vi "Tear Down TS.vi"(8 "error in (no error)":errorcluster, 11 "LNG Boiling Test Stand in":refnum<class "Water Tunnel Test Stand.lvclass">) -> (0 "error out":errorcluster, 3 "LNG Boiling Test Stand out":refnum<class "Water Tunnel Test Stand.lvclass">)   [LabVIEW 2019, in "Test Stands.lvlib" / "Water Tunnel Test Stand.lvclass"]
uses:
  Water Tunnel Test Stand.lvclass
  Water Tunnel Test Stand.lvclass/Water Tunnel Test Stand.ctl
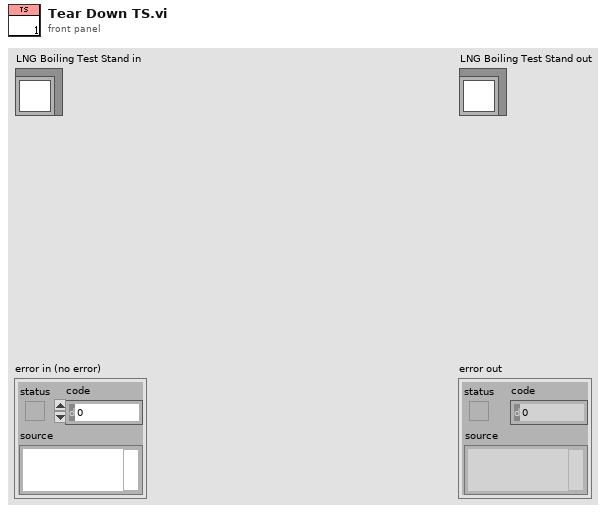
[diagram p1: front panel]
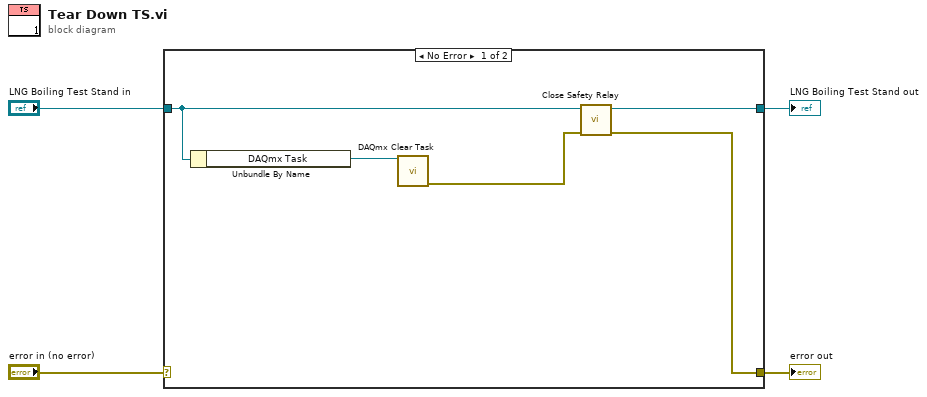
[diagram p0: block diagram]
diagram:
  n1 = case shown="No Error" "error in (no error)" {
    selector: "error in (no error)" -> [_ w11]
    tunnel: [w8 w11] -> w4
    tunnel: [w9 w10] -> w3
    tunnel: "LNG Boiling Test Stand in" -> [w7 w10]
    frame No Error {
      n2 = Unbundle By Name(w7) -> ("DAQmx Task"=w6:refnum<k21>)
      n3 = call <vilib>:"DAQmx Clear Task.vi"("task in"=w6) -> ("error out"=w5:errorcluster)  [unwired: 14 in]
      n4 = call "Close Safety Relay.vi"("error in (no error)"=w5, "LNG Boiling Test Stand in"=w7) -> ("error out"=w8:errorcluster, "LNG Boiling Test Stand out"=w9:refnum<class "Water Tunnel Test Stand.lvclass">)  [unwired: 8 in]
    }
    frame Error {
    }
  }
  "error out" <- w4
  "LNG Boiling Test Stand out" <- w3
